vi "Write Name.vi"(10 "Name":string, 11 "RetentionPolicy in":refnum<class "RetentionPolicy.lvclass">) -> (3 "RetentionPolicy out":refnum<class "RetentionPolicy.lvclass">)   [LabVIEW 2018, in "InfluxDB Client.lvlib" / "RetentionPolicy.lvclass"]
uses:
  RetentionPolicy.lvclass
  RetentionPolicy.lvclass/RetentionPolicy.ctl
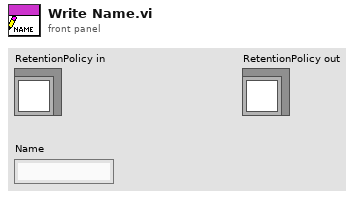
[diagram p1: front panel]
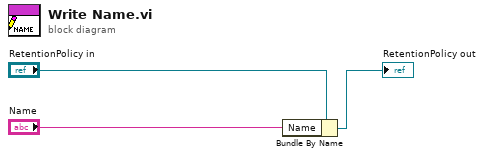
[diagram p0: block diagram]
diagram:
  n1 = Bundle By Name(cluster="RetentionPolicy in", "Name"="Name") -> (→"RetentionPolicy out":refnum<class "RetentionPolicy.lvclass">)
